vi "PH_Sixpack.ProcEvents.vi"(0 "i ref in":refnum<vi>, 5 "error in":errorcluster) -> (14 "i ref out":refnum<vi>, 19 "error out":errorcluster)   [LabVIEW 2014, in "PH_Sixpack.lvlib"]
doc: "This method is used during the 1st frame of the process object to define the events the object will listen to. Add your own events here."
uses:
  PH_Sixpack.lvlib
  CSCore/BaseProcess/BaseProcess.event definition.ctl
  CSCore/CAEObj/CAEObj.event definition.ctl
  CSCore/BaseProcess/BaseProcess.descriptor string definition.ctl
  CSCore/BaseProcess/BaseProcess.lvlib
  CSCore/CAEObj/CAEObj.lvlib
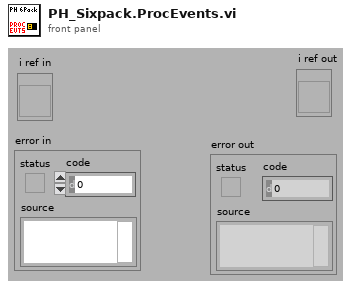
[diagram p1: front panel]
types:
  T1 = typedef "BaseProcess.lvlib/BaseProcess.event definition.ctl" = cluster{"CAEEvtDef":T2, "Data Descriptor":T3}
  T2 = typedef "CAEObj.lvlib/CAEObj.event definition.ctl" = cluster{"URL":string, "enable":bool, "ignoreResID":bool}
  T3 = typedef "BaseProcess.lvlib/BaseProcess.descriptor string definition.ctl" = string
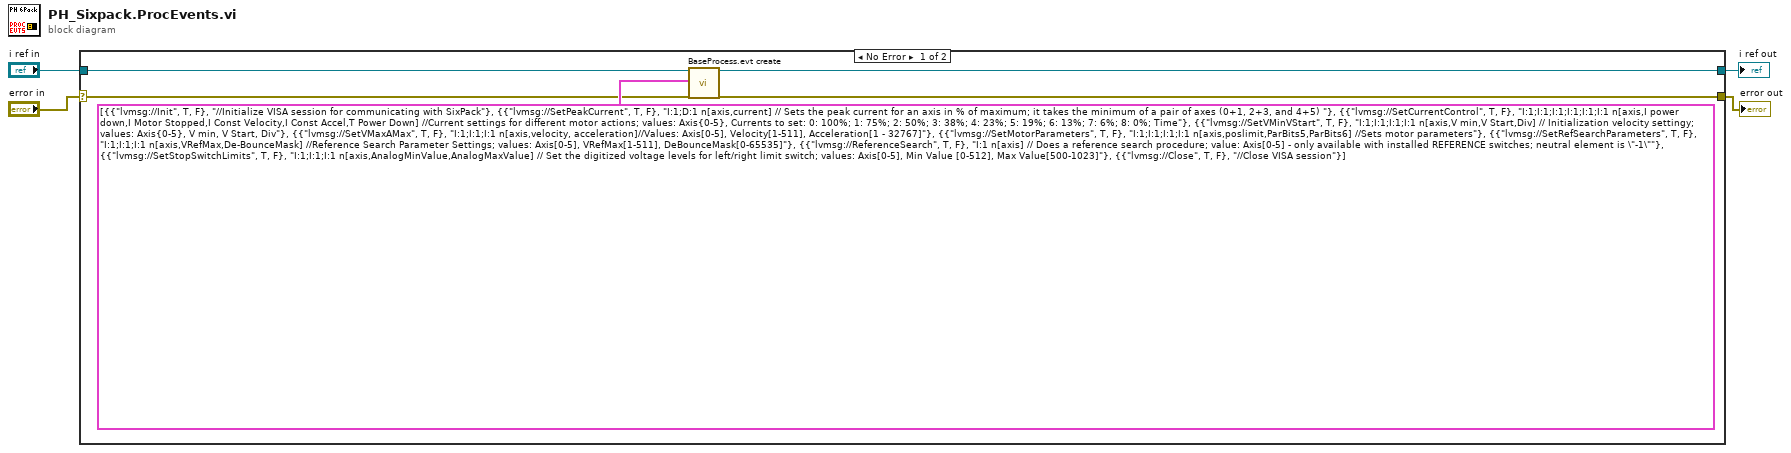
[diagram p0: block diagram]
diagram:
  n1 = case shown="No Error" "error in" {
    selector: "error in" -> [w5 w11]
    tunnel: "i ref in" -> [w6 w10]
    tunnel: [w9 w10] -> w3
    tunnel: [w8 w11] -> w2
    frame No Error {
      n2 = call "BaseProcess.evt create.vi"("i ref in"=w6, "newEvents"=T1[] [{"CAEEvtDef"={"URL"="lvmsg://Init", "enable"=TRUE, "ignoreResID"=FALSE}, "Data Descriptor"="//Initialize VISA session for communicating with SixPack"}, {"CAEEvtDef"={"URL"="lvmsg://SetPeakCurrent", "enable"=TRUE, "ignoreResID"=FALSE}, "Data Descriptor"="I:1;D:1 n[axis,current] // Sets the peak current for an axis in % of maximum; it takes the minimum of a pair of axes (0+1, 2+3, and 4+5) "}, {"CAEEvtDef"={"URL"="lvmsg://SetCurrentControl", "enable"=TRUE, "ignoreResID"=FALSE}, "Data Descriptor"="I:1;I:1;I:1;I:1;I:1;I:1 n[axis,I power down,I Motor Stopped,I Const Velocity,I Const Accel,T Power Down] //Current settings for different motor actions; values: Axis{0-5}, Currents to set: 0: 100%; 1: 75%; 2: 50%; 3: 38%; 4: 23%; 5: 19%; 6: 13%; 7: 6%; 8: 0%; Time"}, {"CAEEvtDef"={"URL"="lvmsg://SetVMinVStart", "enable"=TRUE, "ignoreResID"=FALSE}, "Data Descriptor"="I:1;I:1;I:1;I:1 n[axis,V min,V Start,Div] // Initialization velocity settingy; values: Axis{0-5}, V min, V Start, Div"}, {"CAEEvtDef"={"URL"="lvmsg://SetVMaxAMax", "enable"=TRUE, "ignoreResID"=FALSE}, "Data Descriptor"="I:1;I:1;I:1 n[axis,velocity, acceleration]//Values: Axis[0-5], Velocity[1-511], Acceleration[1 - 32767]"}, {"CAEEvtDef"={"URL"="lvmsg://SetMotorParameters", "enable"=TRUE, "ignoreResID"=FALSE}, "Data Descriptor"="I:1;I:1;I:1;I:1 n[axis,poslimit,ParBits5,ParBits6] //Sets motor parameters"}, {"CAEEvtDef"={"URL"="lvmsg://SetRefSearchParameters", "enable"=TRUE, "ignoreResID"=FALSE}, "Data Descriptor"="I:1;I:1;I:1 n[axis,VRefMax,De-BounceMask] //Reference Search Parameter Settings; values: Axis[0-5], VRefMax[1-511], DeBounceMask[0-65535]"}, {"CAEEvtDef"={"URL"="lvmsg://ReferenceSearch", "enable"=TRUE, "ignoreResID"=FALSE}, "Data Descriptor"="I:1 n[axis] // Does a reference search procedure; value: Axis[0-5] - only available with installed REFERENCE switches; neutral element is \"-1\""}, {"CAEEvtDef"={"URL"="lvmsg://SetStopSwitchLimits", "enable"=TRUE, "ignoreResID"=FALSE}, "Data Descriptor"="I:1;I:1;I:1 n[axis,AnalogMinValue,AnalogMaxValue] // Set the digitized voltage levels for left/right limit switch; values: Axis[0-5], Min Value [0-512], Max Value[500-1023]"}, {"CAEEvtDef"={"URL"="lvmsg://Close", "enable"=TRUE, "ignoreResID"=FALSE}, "Data Descriptor"="//Close VISA session"}] ("appended array"), "error in (no error)"=w5) -> ("i ref out"=w9:refnum<vi>, "error out"=w8:errorcluster)  [unwired: 13 in, 2 out]
    }
    frame Error {
    }
  }
  "i ref out" <- w3
  "error out" <- w2
